vi "String - Format Commands for TSV Output.vi"(8 "Description":string[](array[string]), 9 "Write Access":bool[](array[boolean]), 10 "Read Access":bool[](array[boolean]), 11 "Command":string[](array[string])) -> (3 "Formatted Array":string[][](array[string]))   [LabVIEW 2017, in "Communications Library.lvlib"]
doc: "Used to prepare command information for output to a tab seperated values file.\n\nPrepares a formatted 2D string array of; \n-Command\n-Read Access Property\n-Wire Access Property \n-Command Description"
uses:
  Communications Library.lvlib
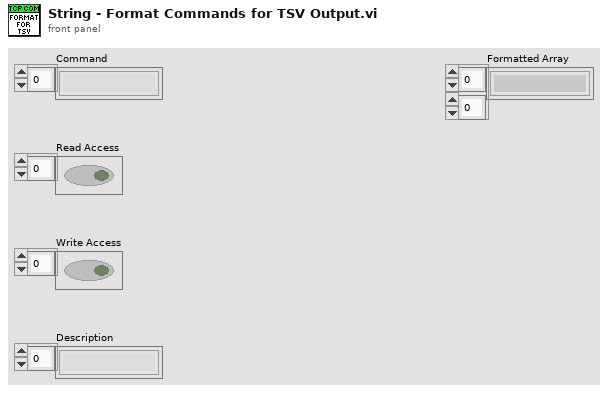
[diagram p1: front panel]
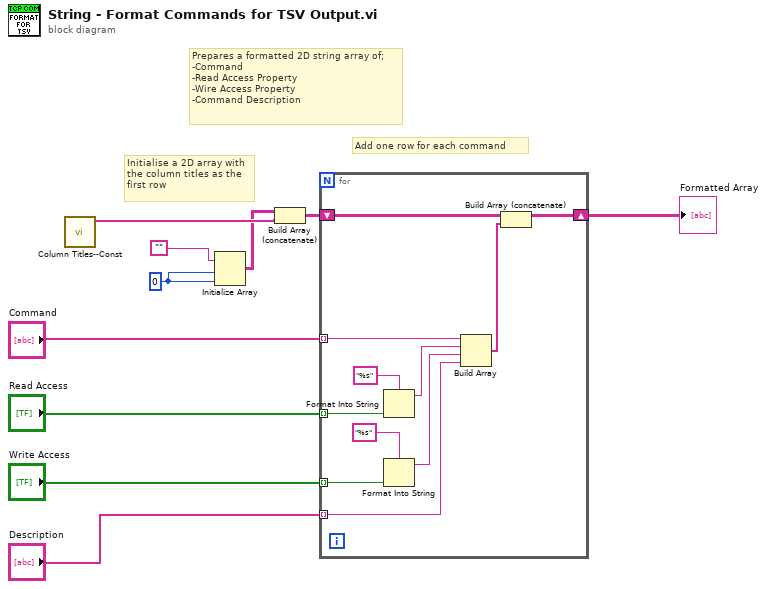
[diagram p0: block diagram]
diagram:
  w1 = 0 ("dimension size")
  # "Prepares a formatted 2D string array of; \n-Command\n-Read Access Property\n-Wire Access Property \n-Command Description"
  # "Add one row for each command"
  # "Initialise a 2D array with\nthe column titles as the \nfirst row"
  n1 = call "Column Titles--Const.vi"() -> ("Column Titles"=w4:string[])  [unwired: 11 in]
  n2 = Initialize Array("", w1, w1) -> (w3:string[][])
  n3 = Build Array (concatenate)(w3, w4) -> (w5:string[][])
  n4 = for {
    shift-right: [w11] -> w10
    shift-left: w5 -> [w13]
    tunnel: "Read Access" -> [w21] mode=indexing
    tunnel: "Write Access" -> [w18] mode=indexing
    tunnel: "Command" -> [w17] mode=indexing
    tunnel: "Description" -> [w14] mode=indexing
    n5 = Format Into String(format string="%s", w21) -> (resulting string=w16:string)  [unwired: 2 in, 1 out]
    n6 = Format Into String(format string="%s", w18) -> (resulting string=w15:string)  [unwired: 2 in, 1 out]
    n7 = Build Array(w17, w16, w15, w14) -> (w12:string[])
    n8 = Build Array (concatenate)(w13, w12) -> (w11:string[][])
  }
  "Formatted Array" <- w10
